vi "queryArtStatus.vi"() -> (0 "采集卡状态":bool)   [LabVIEW 2018]
uses:
  PCI8552B_32.dll
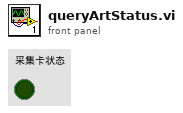
[diagram p1: front panel]
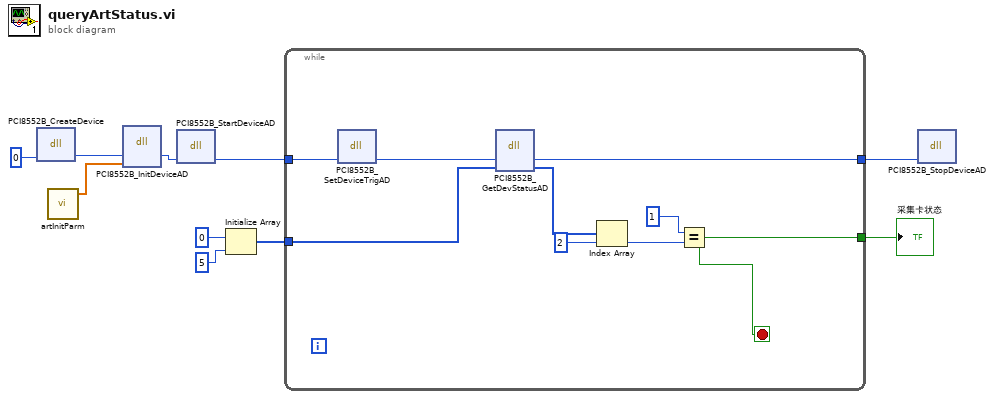
[diagram p0: block diagram]
diagram:
  n1 = dll-call lib="C:/Users/BlueMess/Desktop/Work2020/MMW Controller/mmw_controller/PCI8552B_32.dll" fn="PCI8552B_CreateDevice" label="CreateDevice"("DeviceLgcID"=0) -> ("DeviceLgcID"=w3:i32)  [unwired: 4 in, 2 out]
  n2 = call "artInitParm.vi"() -> ("初始化参数"=w4:dbl[])  [unwired: 2 out]
  n3 = dll-call lib="C:/Users/BlueMess/Desktop/Work2020/MMW Controller/mmw_controller/PCI8552B_32.DLL" fn="PCI8552B_InitDeviceAD" label="InitDeviceAD"("hDevice"=w3, "pADPara"=w4) -> ("hDevice"=w2:i32)  [unwired: 5 in, 2 out]
  n4 = dll-call lib="C:/Users/BlueMess/Desktop/Work2020/MMW Controller/mmw_controller/PCI8552B_32.DLL" fn="PCI8552B_StartDeviceAD" label="StartDeviceAD"("hDevice"=w2) -> ("hDevice"=w5:i32)  [unwired: 4 in, 2 out]
  n5 = Initialize Array(0, 5) -> (w9:i32[])
  n6 = while {
    tunnel: w5 -> [w14]
    tunnel: w9 -> [w19]
    tunnel: [w12] -> w6
    tunnel: [w11] -> w1
    stop <- w11 stop-if-true
    n7 = dll-call lib="C:/Users/BlueMess/Desktop/Work2020/MMW Controller/mmw_controller/PCI8552B_32.DLL" fn="PCI8552B_SetDeviceTrigAD" label="SetDeviceTrigAD"("hDevice"=w14) -> ("hDevice"=w13:i32)  [unwired: 4 in, 2 out]
    n8 = dll-call lib="C:/Users/BlueMess/Desktop/Work2020/MMW Controller/mmw_controller/PCI8552B_32.DLL" fn="PCI8552B_GetDevStatusAD" label="GetDevStatusAD"("hDevice"=w13, "ADStatus"=w19) -> ("hDevice"=w12:i32, "ADStatus"=w15:i32[])  [unwired: 4 in, 2 out]
    n9 = Index Array(array=w15, index=2) -> (element=w17:i32)
    n10 = Equal?(x=1, y=w17) -> (x = y?=w11:bool)
  }
  "采集卡状态" <- w1
  n11 = dll-call lib="C:/Users/BlueMess/Desktop/Work2020/MMW Controller/mmw_controller/PCI8552B_32.DLL" fn="PCI8552B_StopDeviceAD" label="StopDeviceAD"("hDevice"=w6) -> ()  [unwired: 5 in, 2 out]
